vi "Stream_1channel.vi"() -> ()   [LabVIEW 2014]
uses:
  <vilib>/FPGAPlugInAG/PXI-7852R/niLvFpga_Open_PXI-7852R.vi
  <vilib>/rvi/interface/common/dynamic/niFpgaDynamicAddResources.vi
  <vilib>/Utility/error.llb/Error Cluster From Error Code.vi
  <vilib>/rvi/errors/niLvFpgaAdjustHostInterfaceError.vi
  <vilib>/measure/maspectr.llb/FFT Power Spectrum and PSD for 1 Chan.vi
  <vilib>/Utility/file.llb/Write To Spreadsheet File (I64).vi
  <vilib>/FPGAPlugInAG/Dynamic/niLvFpga_Close_Dynamic.vi
  <vilib>/rvi/interface/nirviOpenFPGA/nirviOpenFPGA.xnode
  FPGA Bitfiles/MilitaruDAQ_FPGATarget_Acquisition1chan_k4D6bgHQOE0.lvbitx
  Acquisition_1channel.vi
  <vilib>/rvi/interface/nirviMethod/nirviMethod.xnode
  <vilib>/rvi/interface/nirviCloseFPGA/nirviCloseFPGA.xnode
  <vilib>/FPGAPlugInAG/Dynamic/niLvFpga_ReadFifo_Dynamic.vi
  <vilib>/rvi/errors/niLvFpgaMergeErrorWithErrorCode.vi
  <vilib>/measure/NI_MAPro.lvlib
panel:
  in  "append to file? (new file:F)":bool
  in  "file path (dialog if empty)":path
  out "PSD":cluster{"f0":dbl, "df":dbl, "magnitude":dbl[]}(graph) caption="Dynamic Data Type"
  in  "averaging parameters":T1={"averaging mode"=enum."No averaging", "weighting mode"=enum."Exponential", "number of averages"=10} {"number of averages" min=1}
  in  "dB On (F)":bool
  out "Position":waveform(i16)(graph) caption="Dynamic Data Type"
  in  "Number of Elements":u32
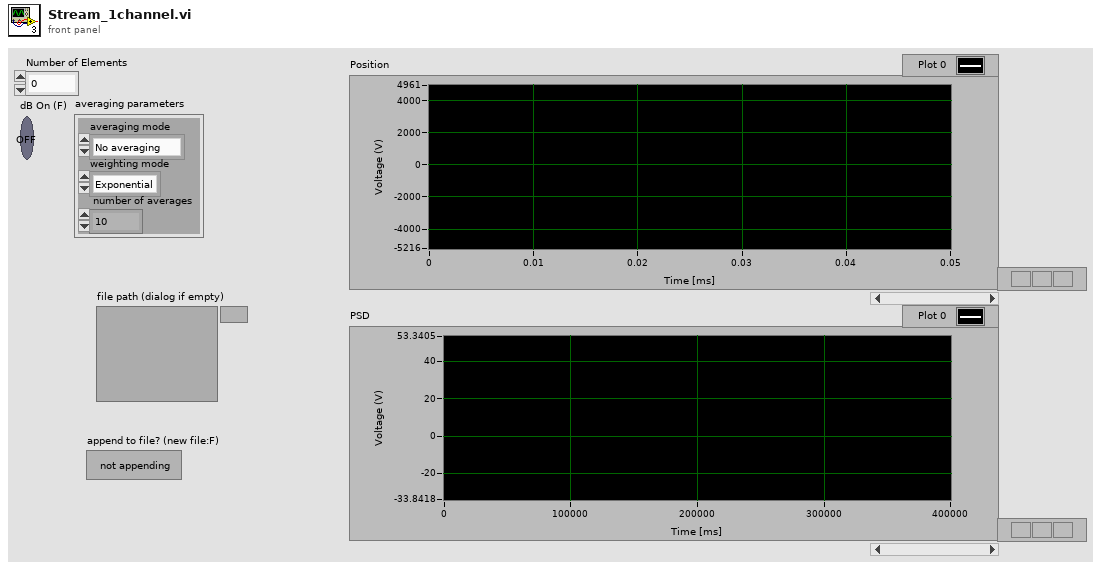
[diagram p1: front panel]
types:
  T1 = cluster{"averaging mode":enum16{"No averaging", "Vector averaging", "RMS averaging", "Peak hold"}, "weighting mode":enum16{"Linear", "Exponential"}, "number of averages":u32}
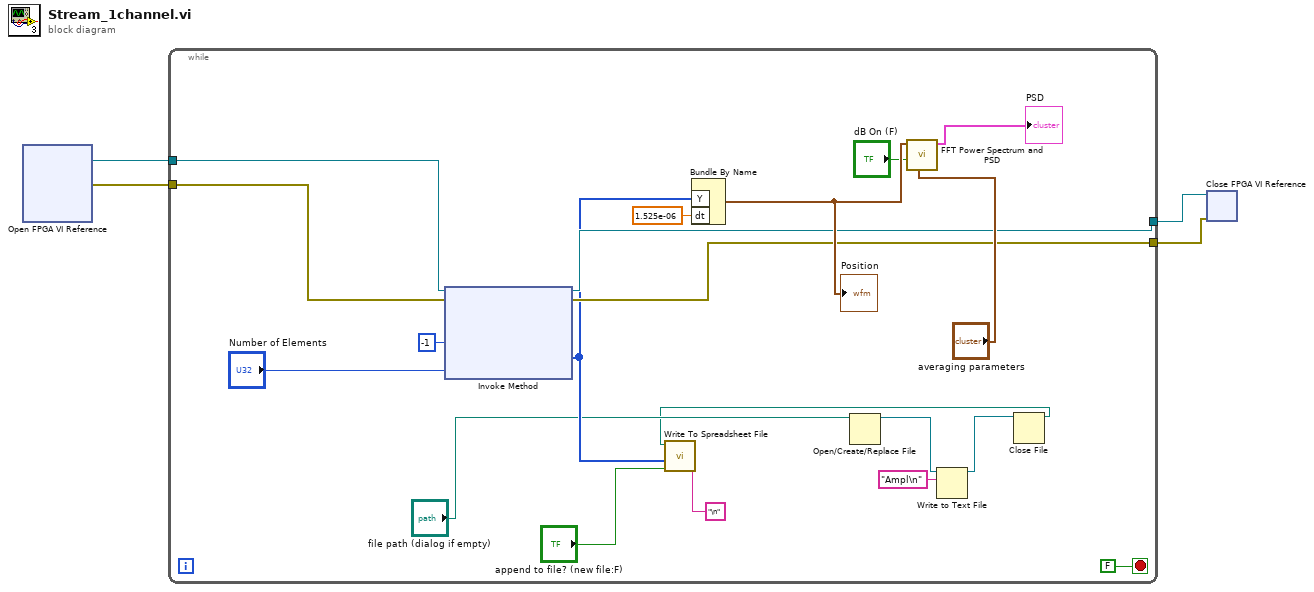
[diagram p0: block diagram]
diagram:
  n1 = xnode "Open FPGA VI Reference"() -> ("FPGA VI Reference Out"=w4:refnum<k20>, "error out"=w3:errorcluster)  [unwired: 2 in]
  n2 = while {
    tunnel: w4 -> [w23]
    tunnel: w3 -> [w22]
    tunnel: [w14] -> w1
    tunnel: [w13] -> w2
    stop <- FALSE stop-if-true
    n3 = xnode "Invoke Method"("FPGA VI Reference In"=w23, "error in"=w22, "Number of Elements"="Number of Elements", "Timeout (ms)"=-1) -> ("FPGA VI Reference Out"=w14:refnum<k20>, "error out"=w13:errorcluster, "Data"=w12:i16[])  [unwired: 1 out]
    n4 = Bundle By Name ("Build Waveform")("Y"=w12, "dt"=1.525e-06) -> (w18:waveform(i16))  [unwired: 1 in]
    "Position" <- w18
    n5 = Open/Create/Replace File(file path (use dialog)="file path (dialog if empty)") -> (refnum out=w8:refnum<file>)  [unwired: 5 in, 2 out]
    n6 = call-poly <vilib>:"FFT Power Spectrum and PSD.vi"("averaging parameters"="averaging parameters", "dB On (F)"="dB On (F)", "time signal"=w18) -> ("Power Spectrum / PSD"=→"PSD":cluster{"f0":dbl, "df":dbl, "magnitude":dbl[]})  [unwired: 5 in, 3 out]
    n7 = Write to Text File(file (use dialog)=w8, text="Ampl\n") -> (refnum out=w7:refnum<file>)  [unwired: 2 in, 2 out]
    n8 = Close File(refnum=w7) -> (path=w6:path)  [unwired: 1 in, 1 out]
    n9 = call-poly <vilib>:"Write To Spreadsheet File.vi"("delimiter (\\t)"="\n" ("delimiter (\\t)"), "append to file? (new file:F)"="append to file? (new file:F)", "1D data"=w12, "file path (dialog if empty)"=w6) -> ()  [unwired: 4 in, 1 out]
  }
  n10 = xnode "Close FPGA VI Reference"("FPGA VI Reference In"=w1, "error in"=w2) -> ()  [unwired: 1 out]
